vi "Initialize-SM1000.vi"(8 "error in (no error)":errorcluster, 11 "Data ref. in":T1) -> (0 "error out":errorcluster, 3 "Data ref.":T1)   [LabVIEW 2013, in "HardwareCharacterization.lvlib" / "HC-Main.lvclass"]
uses:
  HC-Main.lvclass
  Object-reference.ctl
  SM1000/TCP-settings.ctl
  SM1000/DOTNET-settings.ctl
  SM1000/Device-identification.ctl
  HC-Main.lvclass/HC-Main.ctl
  SM1000/HC-SM1000.lvclass
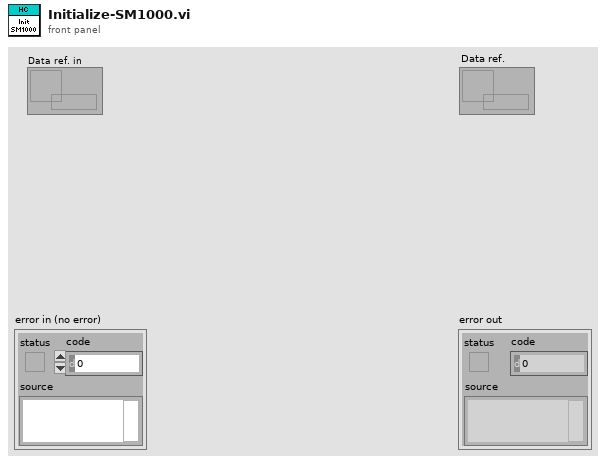
[diagram p1: front panel]
types:
  T1 = typedef "HardwareCharacterization.lvlib/HC-Main.lvclass/Object-reference.ctl" = refnum<data-value>
  T2 = typedef "HardwareCharacterization.lvlib/HC-SM1000.lvclass/DOTNET-settings.ctl" = cluster{"Target IP":string, "Target broadcast port":i32, "Target communication port":i32, "clientID":i32, "Broadcast IP":string, "Servercount":i32, "Device IDs":T3[]}
  T3 = typedef "HardwareCharacterization.lvlib/HC-SM1000.lvclass/Device-identification.ctl" = cluster{"Name":string, "IP":string, "Mac address":string}
  T4 = typedef "HardwareCharacterization.lvlib/HC-SM1000.lvclass/TCP-settings.ctl" = cluster{"Target IP":string, "Target TCP port":u16, "TCP read mode":enum16{"Standard", "Buffered", "CRLF", "Immediate"}, "TCP read buffer":i32, "Read timeout":i32}
  T5 = typedef "HardwareCharacterization.lvlib/HC-SM1000.lvclass/Object-reference.ctl" = refnum<data-value>
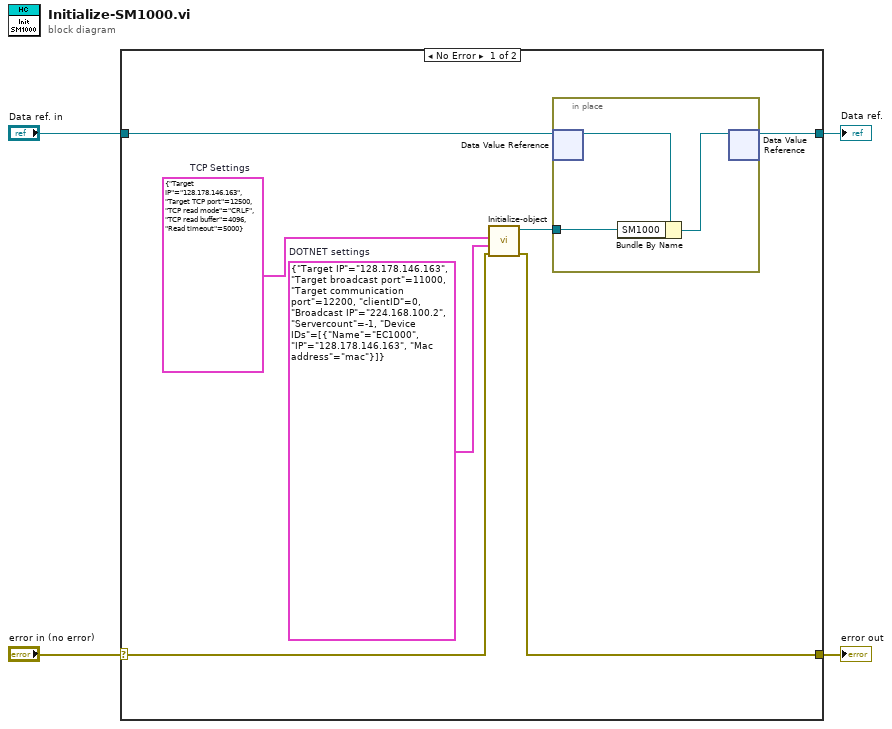
[diagram p0: block diagram]
diagram:
  n1 = case shown="No Error" "error in (no error)" {
    selector: "error in (no error)" -> [w8 w16]
    tunnel: [w7 w16] -> w3
    tunnel: "Data ref. in" -> [w10 w15]
    tunnel: [w11 w15] -> w1
    frame No Error {
      w5 = T2 {"Target IP"="128.178.146.163", "Target broadcast port"=11000, "Target communication port"=12200, "clientID"=0, "Broadcast IP"="224.168.100.2", "Servercount"=-1, "Device IDs"=[{"Name"="EC1000", "IP"="128.178.146.163", "Mac address"="mac"}]}  # DOTNET settings
      w6 = T4 {"Target IP"="128.178.146.163", "Target TCP port"=12500, "TCP read mode"=enum."CRLF", "TCP read buffer"=4096, "Read timeout"=5000}  # TCP Settings
      n2 = call "Initialize-object.vi"("error in (no error)"=w8, "DOTNET settings"=w5, "TCP settings"=w6) -> ("error out"=w7:errorcluster, "SM1000-control out"=w9:T5)  [unwired: 7 in]
      n3 = in-place {
        in-place-border: w9 -> [w14]
        n4 = in-place-dvr #1(w10) -> (w12:refnum<class "HC-Main.lvclass">)  [unwired: 1 out]
        n5 = Bundle By Name(cluster=w12, "SM1000"=w14) -> (w13:refnum<class "HC-Main.lvclass">)
        n6 = in-place-dvr #1(w13) -> (w11:T1)  [unwired: 1 out]
      }
    }
    frame Error {
    }
  }
  "error out" <- w3
  "Data ref." <- w1
